vi "E441X_PM_Set_Initiate_Continuous_State.vi"(0 "VISA session":refnum<visa-resource-name>, 1 "Channel (0: A)":i32(ring) items=["A", "B"], 5 "State (T: On)":bool=TRUE, 11 "error in (no error)":errorcluster {"code" format="%.0x"}) -> (4 "dup VISA session":refnum<visa-resource-name>, 15 "error out":errorcluster {"code" format="%.0x"})   [LabVIEW 2015]
doc: "This VI sets the power meter for continuous trigger cycles."
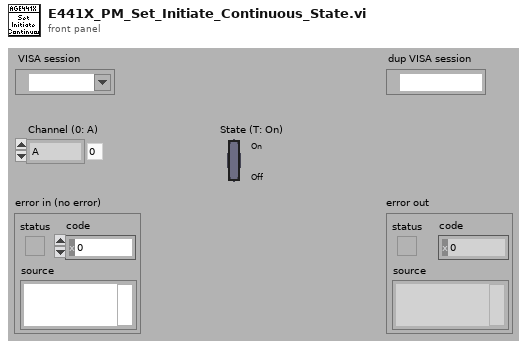
[diagram p1: front panel]
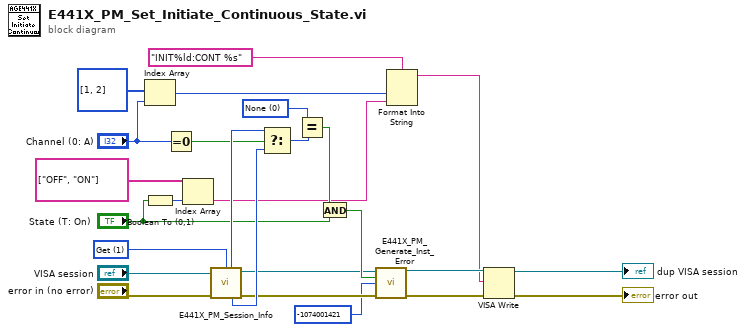
[diagram p0: block diagram]
diagram:
  w19 = 0 items=["None", "8480", "E Series", "E9320"] ("Sensor A (0: None)")
  w24 = 1 items=["Set", "Get"] ("Operation")
  n1 = Index Array(array=i32[] [1, 2], index="Channel (0: A)") -> (element=w2:i32)
  n2 = Boolean To (0,1)(Boolean="State (T: On)") -> (0, 1=w11:i16)
  n3 = Equal To 0?(x="Channel (0: A)") -> (x = 0?=w22:bool)
  n4 = Index Array(array=string[] ["OFF", "ON"], index=w11) -> (element=w7:string)
  n5 = call "E441X_PM_Session_Info.vi"("VISA session"="VISA session", "Operation"=w24, "error in (no error)"="error in (no error)") -> ("Sensor A (0: None)"=w23:i32, "dup VISA session"=w17:refnum<visa-resource-name>, "Sensor B (0: None)"=w21:i32, "error out"=w16:errorcluster)  [unwired: 7 in, 2 out]
  n6 = Select(t=w23, s=w22, f=w21) -> (s? t:f=w20:i32)
  n7 = Equal?(x=w19, y=w20) -> (x = y?=w12:bool)
  n8 = And(x=w12, y="State (T: On)") -> (x .and. y?=w18:bool)
  n9 = call "E441X_PM_Generate_Inst_Error.vi"("VISA session"=w17, "Error State (F: Off)"=w18, "Code (0 - No error)"=-1074001421, "error in (no error)"=w16) -> ("dup VISA session"=w9:refnum<visa-resource-name>, "error out"=w8:errorcluster)  [unwired: 10 in]
  n10 = Format Into String(format string="INIT%ld:CONT %s", w2, w7) -> (resulting string=w6:string)  [unwired: 2 in, 1 out]
  n11 = VISA Write(VISA resource name=w9, write buffer=w6, error in (no error)=w8) -> (VISA resource name out=→"dup VISA session":refnum<visa-resource-name>, error out=→"error out":errorcluster)  [unwired: 1 out]
